vi "refnums.vi"() -> ()   [LabVIEW 2019]
panel:
  out "Test Solenoid":string
  out "Pressure_Transducer":string
  out "Beam_Break_0":string
  out "Joystick_Manipulator":string
  out "LED_2":string
  out "LED_1":string
  out "Wheel_3_Pot":string
  out "Wheel_2_Pot":string
  out "Wheel_1_Pot":string
  out "Wheel_0_Pot":string
  out "Wheel_3_Azimuth":string
  out "Wheel_2_Azimuth":string
  out "IMU_0":string
  out "Joystick_Driver":string
  out "Compressor":string
  out "Wheel_1_Azimuth":string
  out "Wheel_0_Azimuth":string
  out "Wheel_3_Speed":string
  out "Wheel_2_Speed":string
  out "Wheel_1_Speed":string
  out "Wheel_0_Speed":string
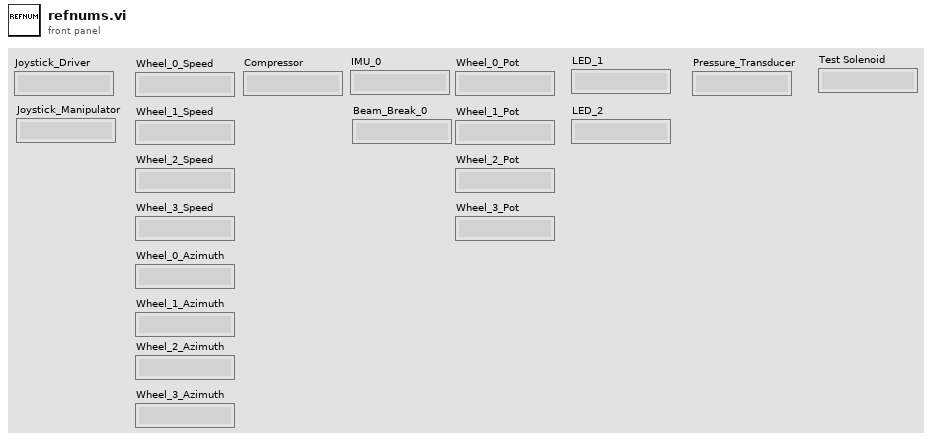
[diagram p1: front panel]
diagram:
